vi "WPI_CameraApplyServerCameraSettings.vi"(9 "Unique":T1, 10 "Additional Settings":T2, 11 "CameraDevRef":T3) -> (2 "Brightness":i32, 3 "CameraDevRef Out":T3)   [LabVIEW 2017]
uses:
  <vilib>/Rock Robotics/WPI/Camera/WPI_CameraDevRef.ctl
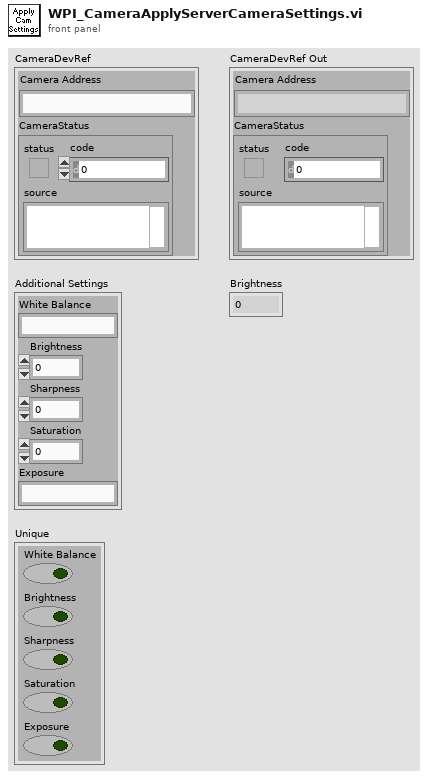
[diagram p1: front panel]
types:
  T1 = cluster{"White Balance":bool, "Brightness":bool, "Sharpness":bool, "Saturation":bool, "Exposure":bool}
  T2 = cluster{"White Balance":string, "Brightness":i32, "Sharpness":i32, "Saturation":i32, "Exposure":string}
  T3 = typedef "WPI_CameraDevRef.ctl" = cluster{"Camera Address":string, "CameraStatus":errorcluster}
  T4 = typedef "WPI_CameraWhite Balance Values.ctl" = enum16{"Auto", "Fixed indoor", "Fixed outdoor 1", "Fixed outdoor 2", "Fixed fluorescent 1", "Fixed fluorescent 2", "Hold current", "Custom"}
  T5 = typedef "WPI_CameraExposure Values.ctl" = enum16{"Auto", "Flicker-free 50 Hz", "Flicker-free 60 Hz", "Hold current", "Custom"}
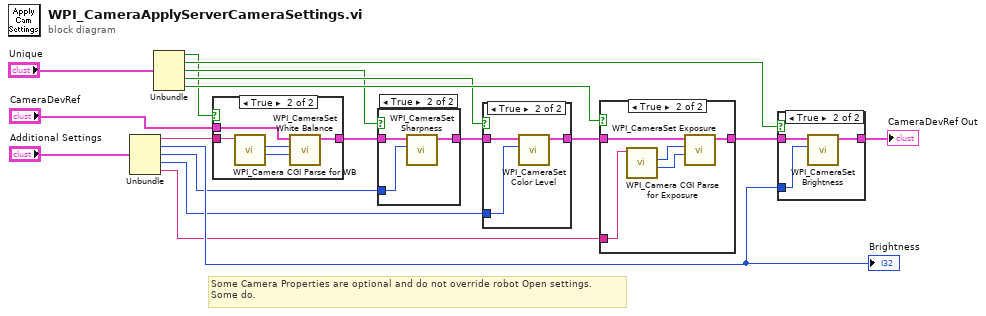
[diagram p0: block diagram]
diagram:
  # "Some Camera Properties are optional and do not override robot Open settings.\nSome do."
  n1 = Unbundle("Additional Settings") -> ("White Balance"=w7:string, "Brightness"=w18:i32, "Sharpness"=w8:i32, "Saturation"=w9:i32, "Exposure"=w10:string)
  "Brightness" <- w18
  n2 = Unbundle("Unique") -> ("White Balance"=w3:bool, "Brightness"=w16:bool, "Sharpness"=w4:bool, "Saturation"=w5:bool, "Exposure"=w6:bool)
  n3 = case shown="True" w3 {
    tunnel: "CameraDevRef" -> [w19 w24]
    tunnel: [w19 w23] -> w14
    tunnel: w7 -> [_ w20]
    frame False {
    }
    frame True {
      n4 = call <vilib>:"WPI_Camera CGI Parse for WB.vi"("String"=w20) -> ("Numeric"=w21:i32, "enum"=w22:T4)  [unwired: 9 in]
      n5 = call <vilib>:"WPI_CameraSet White Balance.vi"("Color Temp (K)"=w21, "White Balance"=w22, "CameraDevRef"=w24) -> ("CameraDevRef Out"=w23:T3)  [unwired: 7 in, 1 out]
    }
  }
  n6 = case shown="True" w4 {
    tunnel: w14 -> [w25 w28]
    tunnel: [w25 w27] -> w12
    tunnel: w8 -> [_ w26]
    frame False {
    }
    frame True {
      n7 = call <vilib>:"WPI_CameraSet Sharpness.vi"("Sharpness"=w26, "CameraDevRef"=w28) -> ("CameraDevRef Out"=w27:T3)  [unwired: 8 in, 1 out]
    }
  }
  n8 = case shown="True" w5 {
    tunnel: w12 -> [w29 w32]
    tunnel: [w29 w31] -> w13
    tunnel: w9 -> [_ w30]
    frame False {
    }
    frame True {
      n9 = call <vilib>:"WPI_CameraSet Color Level.vi"("Color Level"=w30, "CameraDevRef"=w32) -> ("CameraDevRef Out"=w31:T3)  [unwired: 8 in, 1 out]
    }
  }
  n10 = case shown="True" w6 {
    tunnel: w13 -> [w33 w38]
    tunnel: [w33 w37] -> w15
    tunnel: w10 -> [_ w36]
    frame False {
    }
    frame True {
      n11 = call <vilib>:"WPI_Camera CGI Parse for Exposure.vi"("String"=w36) -> ("Numeric"=w35:i32, "enum"=w34:T5)  [unwired: 9 in]
      n12 = call <vilib>:"WPI_CameraSet Exposure.vi"("Exposure (%)"=w35, "Exposure"=w34, "CameraDevRef"=w38) -> ("CameraDevRef Out"=w37:T3)  [unwired: 7 in, 1 out]
    }
  }
  n13 = case shown="True" w16 {
    tunnel: w15 -> [w39 w42]
    tunnel: [w39 w41] -> w17
    tunnel: w18 -> [_ w40]
    frame False {
    }
    frame True {
      n14 = call <vilib>:"WPI_CameraSet Brightness.vi"("Brightness"=w40, "CameraDevRef"=w42) -> ("CameraDevRef Out"=w41:T3)  [unwired: 8 in, 1 out]
    }
  }
  "CameraDevRef Out" <- w17
